vi "MainNR.vi"(10 "JQMHStartup":refnum<class "RQMHStartup.lvclass">, 11 "NewTemplate in":refnum<class "Testing.lvclass">) -> ()   [LabVIEW 2024, in "Testing.lvclass"]
uses:
  Testing.lvclass
  C:/Github/JQMH/JQMHCore/Module/RQMHModule.lvclass
  JQMHCore/JQMHStartup/RQMHStartup.lvclass
  Message Queue_class/RQMHMessageQueue.lvclass/RQMHMessageQueue.ctl
  JQMHCore/Module/InitialiseReplyArgs.ctl
  <vilib>/Utility/miscctls.llb/LVPointTypeDef.ctl
  JQMHCore/Module/RQMHModule.lvclass/RQMHModule.ctl
  Do Something ReplyArgs.ctl
  Do Something Args.ctl
  NewRequest ReplyArgs.ctl
  NewRequest Args.ctl
  JQMHCore/Module/Read ModuleName.vi
  JQMHCore/Module/Read External Start.vi
  Message Queue_class/Delacor_lib_QMH_Enqueue Message (Single).vi
  Message Queue_class/RQMHMessageQueue.lvclass
  Testing.lvclass/Testing.ctl
  JQMHCore/Module/RQMHModule.lvclass
  JQMHCore/Shared/JQMHShared.lvlib
panel:
  out "error out":errorcluster
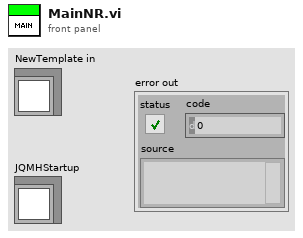
[diagram p1: front panel]
types:
  T1 = typedef "Testing.lvclass/Request Events--cluster.ctl" = cluster{"Do Something":refnum<user-event>, "NewRequest":refnum<user-event>}
  T2 = cluster{"Stop Module":refnum<user-event>, "Requests":T1}
  T3 = typedef "LVPointTypeDef.ctl" = cluster{"Horizontal":i16, "Vertical":i16}
  T4 = enum32{"Invalid", "Standard", "Closed", "Hidden", "Minimized", "Maximized"}
  T5 = typedef "RQMHModule.lvclass/InitialiseReplyArgs.ctl" = cluster{"Did Init?":bool}
  T6 = typedef "Testing.lvclass/Do Something Args.ctl" = cluster{"Msg":string}
  T7 = typedef "Testing.lvclass/Do Something ReplyArgs.ctl" = cluster{"Value":dbl, "Boolean":bool}
  T8 = typedef "Testing.lvclass/NewRequest Args.ctl" = cluster{"String":string}
  T9 = typedef "Testing.lvclass/NewRequest ReplyArgs.ctl" = cluster{"Numeric":dbl}
  T10 = typedef "RQMHModule.lvclass/Reply.ctl" = cluster{"Expects Reply":bool, "Reply":refnum<notifier>}
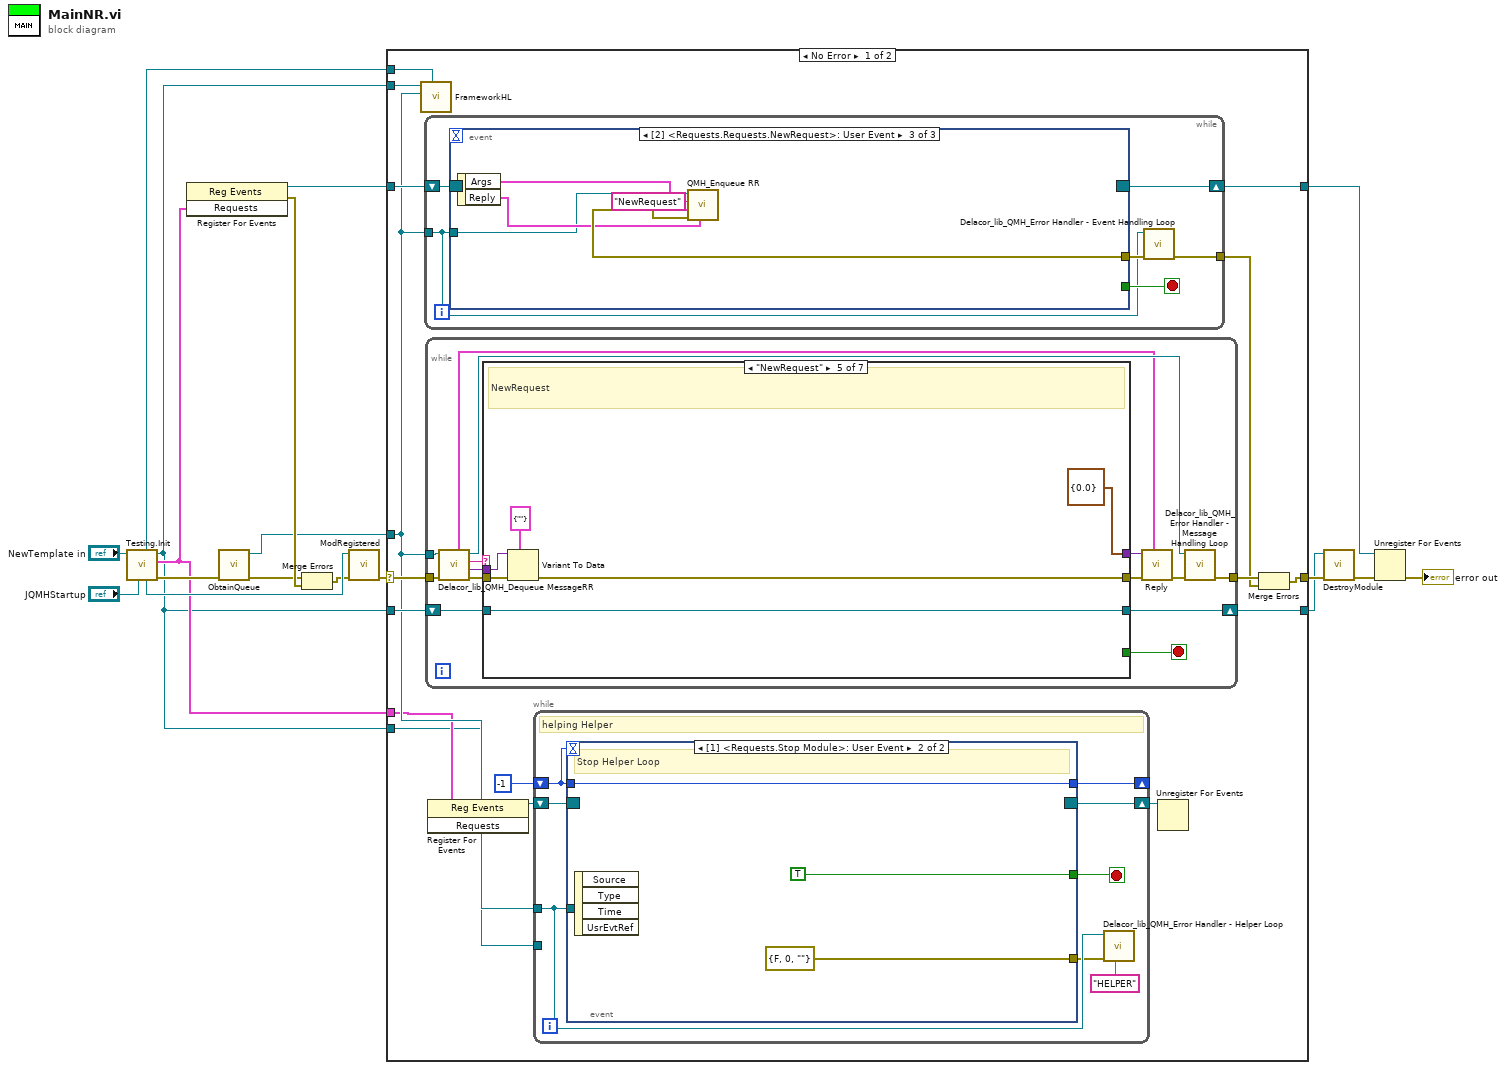
[diagram p0: block diagram]
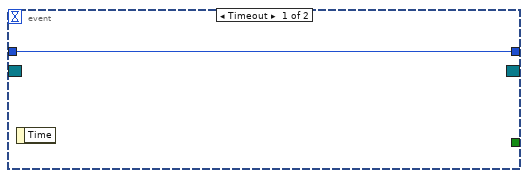
[diagram p2: hidden frame]
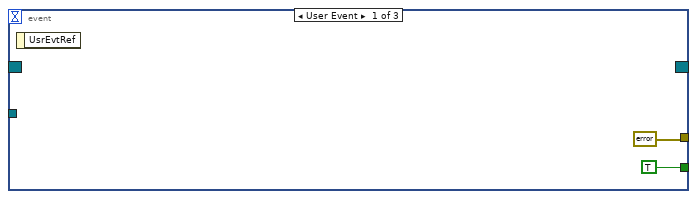
[diagram p3: hidden frame]
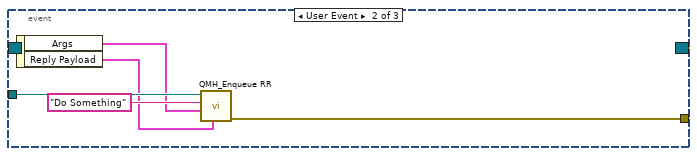
[diagram p4: hidden frame]
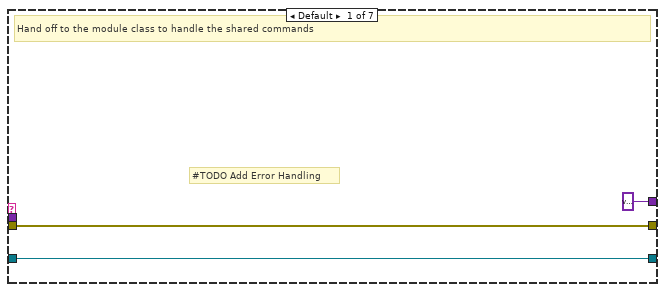
[diagram p5: hidden frame]
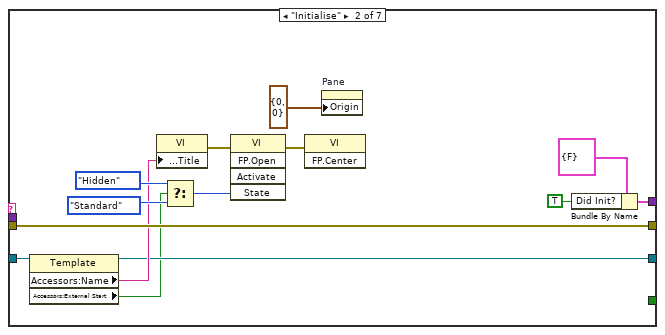
[diagram p6: hidden frame]
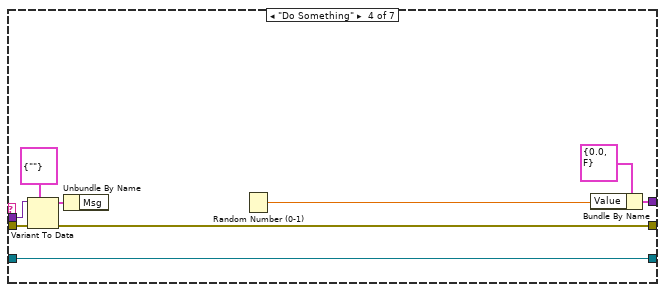
[diagram p8: hidden frame]
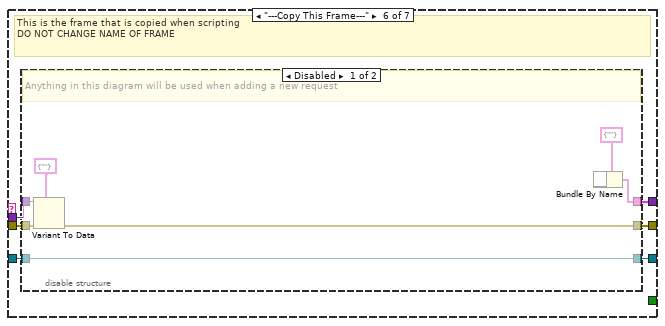
[diagram p9: hidden frame]
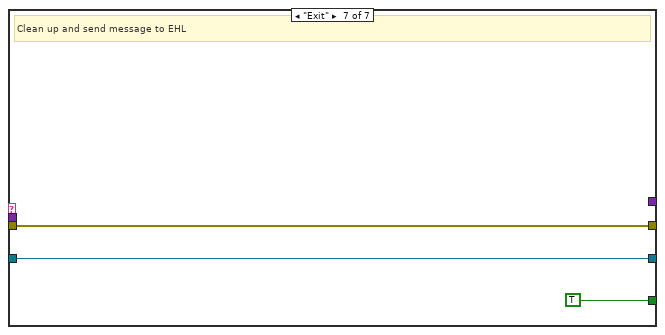
[diagram p11: hidden frame]
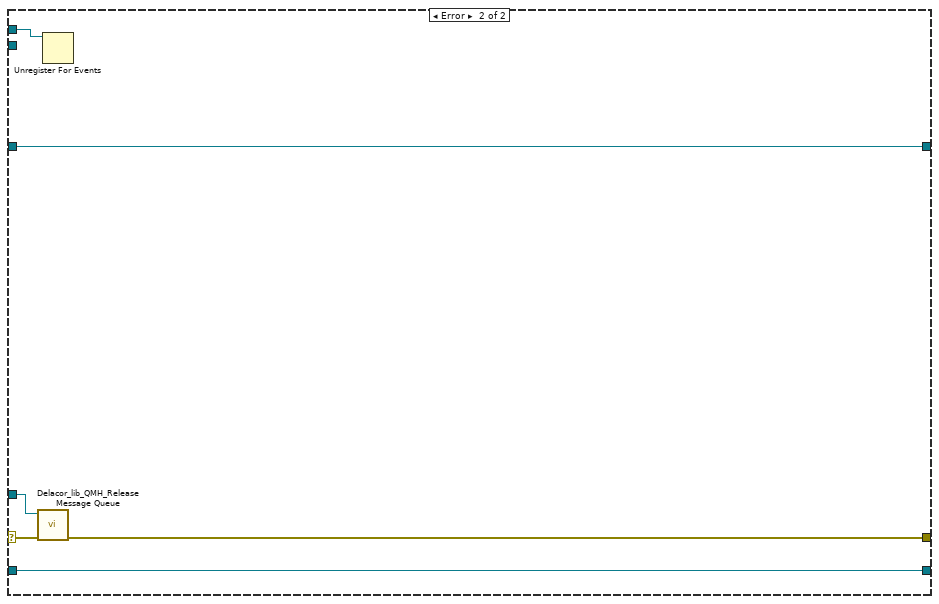
[diagram p12: hidden frame]
diagram:
  n1 = call "Testing.Init.vi"("JQMHStartup in"="JQMHStartup", "NewTemplate in"="NewTemplate in") -> ("error out"=w11:errorcluster, "Requests"=w2:T2, "NewTemplate out"=w1:refnum<class "Testing.lvclass">, "JQMHStartup out"=w9:refnum<class "RQMHStartup.lvclass">, "StandardRequests"=w5:refnum<event-registration>)  [unwired: 4 in, 1 out]
  n2 = register-events(w2) -> (reference out=w4:refnum<event-registration>, error out=w18:errorcluster)  [unwired: 2 in]
  n3 = call "ObtainQueue.vi"("error in"=w11) -> ("error out"=w10:errorcluster, "Message Queue"=w6:refnum<class "RQMHMessageQueue.lvclass">)  [unwired: 9 in]
  n4 = Merge Errors(w10, w18) -> (w7:errorcluster)
  n5 = call "ModRegistered.vi"("error in (no error)"=w7, "JQMHStartup in"=w9) -> ("error out"=w8:errorcluster)  [unwired: 9 in]
  n6 = case "RQMH_MAIN" shown="No Error" w8 {
    selector: w8 -> [w31 w134]
    tunnel: w1 -> [w34 w133]
    tunnel: [w33 w136] -> w17
    tunnel: w4 -> [w32 w136]
    tunnel: w6 -> [w25 w135]
    tunnel: [w30 w133] -> w3
    tunnel: [w27 w132] -> w14
    tunnel: w1 -> [w26 _]
    tunnel: w5 -> [w24 w131]
    tunnel: w2 -> [w23 _]
    tunnel: w1 -> [w22 _]
    frame No Error {
      n7 = call-dynamic "FrameworkHL.vi"("StandardRequests"=w24, "Message Queue"=w25, "JQMHModule in"=w26) -> ()  [unwired: 9 in]
      n8 = while {
        shift-right: [w52] -> w33
        shift-left: w32 -> [w47]
        tunnel: w25 -> [w48]
        tunnel: [w49] -> w28
        stop <- w51 stop-if-true
        n9 = event "RQMH_EVENT_MAIN" shown="[2] <Requests.Requests.NewRequest>: User Event" {
          selector: w47 -> [_ _ _]
          dyn-events: [_ _ _] -> w52
          timeout: _ -> [_ _ _]
          tunnel: [TRUE _ _] -> w51
          tunnel: w48 -> [_ w59 w61]
          tunnel: [errorcluster {"status"=FALSE, "code"=0, "source"=""} ("error out") w56 w64] -> w50
          event User Event {
            n10 = event-data() -> ()  [unwired: 1 in, 1 out]
          }
          event User Event {
            n11 = event-data() -> ("Args"=w57:T6, "Reply Payload"=w55:T10)  [unwired: 1 in]
            n12 = call "QMH_Enqueue RR.vi"("Reply"=w55, "Message Data"=w57, "Message"="Do Something", "Message Queue in"=w59) -> ("error out"=w56:errorcluster)  [unwired: 6 in, 1 out]
          }
          event User Event {
            n13 = event-data() -> ("Args"=w62:T8, "Reply"=w63:T10)  [unwired: 1 in]
            n14 = call "QMH_Enqueue RR.vi"("Reply"=w63, "Message Data"=w62, "Message"="NewRequest", "Message Queue in"=w61) -> ("error out"=w64:errorcluster)  [unwired: 6 in, 1 out]
          }
        }
        n15 = call-dynamic "Delacor_lib_QMH_Error Handler - Event Handling Loop.vi"("error in"=w50, "Message Queue in"=w48) -> ("dup error in"=w49:errorcluster)  [unwired: 8 in, 1 out]
      }
      n16 = while {
        tunnel: w25 -> [w73]
        tunnel: w31 -> [w72]
        shift-right: [w75] -> w30
        shift-left: w34 -> [w76]
        tunnel: [w74] -> w29
        stop <- w78 stop-if-true
        n17 = call-dynamic "Delacor_lib_QMH_Dequeue MessageRR.vi"("error in"=w72, "Message Queue in"=w73) -> ("error out"=w71:errorcluster, "Message Data"=w69:variant, "Message"=w70:string, "Message Queue out"=w77:refnum<class "RQMHMessageQueue.lvclass">, "Reply"=w65:T10)  [unwired: 5 in]
        n18 = case "RQMH_MESSAGE_CASES" shown="\"NewRequest\"" w70 {
          tunnel: [_ _ _ _ _ _ TRUE] -> w78
          tunnel: w76 -> [w80 w83 w96 w106 w110 w116 w129]
          tunnel: w69 -> [_ _ _ w102 w109 w114 _]
          tunnel: w71 -> [w81 w95 w97 w101 w112 w118 w128]
          tunnel: [w81 w95 w97 w100 w111 w117 w128] -> w68
          tunnel: [w80 w84 w96 w106 w110 w115 w129] -> w75
          tunnel: [variant w94 _ w105 T9 {"Numeric"=0.0} ("RQMH_MHL_REPLY_PL") w113 _] -> w66
          frame Default {
            # "#TODO Add Error Handling"
            # "Hand off to the module class to handle the shared commands"
          }
          frame "Initialise" {
            n19 = property class="Template"(reference=w83) -> (reference out=w84:refnum<class "Testing.lvclass">, "Accessors:Name"=w85:string, "Accessors:External Start"=w82:bool)  [unwired: 1 in, 1 out]
            n20 = property on="Property Node" class="VI"("Front Panel.Title"=w85) -> (error out=w92:errorcluster)  [unwired: 2 in, 1 out]
            n21 = Select(t=T4."Hidden" ("State"), s=w82, f=T4."Standard" ("State")) -> (s? t:f=w88:T4)
            n22 = invoke on="Invoke Node" class="VI" method="FP.Open"(error in=w92, "State"=w88) -> (error out=w91:errorcluster)  [unwired: 3 in, 4 out]
            n23 = invoke on="Invoke Node" class="VI" method="FP.Center"(error in=w91) -> ()  [unwired: 2 in, 3 out]
            n24 = property on="Pane" class="Pane"("Origin"=T3 {"Horizontal"=0, "Vertical"=0}) -> ()  [unwired: 2 in, 2 out]
            n25 = Bundle By Name(cluster=T5 {"Did Init?"=FALSE} ("Args"), "Did Init?"=TRUE) -> (w94:T5)
          }
          frame "---Module Specific---" {
          }
          frame "Do Something" {
            n26 = Variant To Data(error in=w101, type=T6 {"Msg"=""} ("Do Something Args"), Variant=w102) -> (data=w98:T6, error out=w100:errorcluster)
            n27 = Unbundle By Name(w98) -> ()  [unwired: 1 out]
            n28 = Random Number (0-1)() -> (number: 0 to 1=w103:dbl)
            n29 = Bundle By Name(cluster=T7 {"Value"=0.0, "Boolean"=FALSE}, "Value"=w103) -> (w105:T7)
          }
          frame "NewRequest" {
            # "NewRequest"
            n30 = Variant To Data(error in=w112, type=T8 {"String"=""} ("RQMH_MHL_MSG_PL"), Variant=w109) -> (error out=w111:errorcluster)  [unwired: 1 out]
          }
          frame "---Copy This Frame---" {
            # "This is the frame that is copied when scripting\nDO NOT CHANGE NAME OF FRAME"
            n31 = disable-structure shown="Disabled" {
              disable-tunnel: w118 -> [w122 w127]
              disable-tunnel: [w123 w127] -> w117
              disable-tunnel: w116 -> [w125 w126]
              disable-tunnel: [w125 w126] -> w115
              disable-tunnel: w114 -> [w124 _]
              disable-tunnel: [w120 _] -> w113
              frame Disabled {
                # "Anything in this diagram will be used when adding a new request"
                n32 = Variant To Data(error in=w122, type=cluster{string} {""} ("RQMH_MHL_MSG_PL"), Variant=w124) -> (error out=w123:errorcluster)  [unwired: 1 out]
                n33 = Bundle By Name(cluster=cluster{string} {""} ("RQMH_MHL_REPLY_PL")) -> (w120:cluster{string})  [unwired: 1 in]
              }
              frame Enabled {
              }
            }
          }
          frame "Exit" {
            # "Clean up and send message to EHL"
          }
        }
        n34 = call "Reply.vi"("Reply"=w65, "error in (no error)"=w68, "ReplyPayload"=w66) -> ("error out"=w67:errorcluster)  [unwired: 8 in]
        n35 = call-dynamic "Delacor_lib_QMH_Error Handler - Message Handling Loop.vi"("error in"=w67, "Message Queue in"=w77) -> ("dup error in"=w74:errorcluster)  [unwired: 8 in, 1 out]
      }
      n36 = register-events ("DQMH_HELPER_REGFOREVENTS")(w23) -> (reference out=w20:refnum<event-registration>)  [unwired: 2 in, 1 out]
      n37 = while "RQMH_HELPER_LOOP" {
        shift-right: [w42] -> _
        shift-left: -1 -> [w41]
        shift-right: [w39] -> w19
        shift-left: w20 -> [w40]
        tunnel: w25 -> [w37]
        tunnel: w22 -> [_]
        stop <- w38 stop-if-true
        # "helping Helper"
        n38 = event "RQMH_HELPER_EVENT_STRUCTURE" shown="[1] <Requests.Stop Module>: User Event" {
          selector: w40 -> [_ _]
          dyn-events: [_ _] -> w39
          timeout: w41 -> [_ _]
          tunnel: w41 -> [w43 w46]
          tunnel: [w43 w46] -> w42
          tunnel: [_ TRUE] -> w38
          tunnel: [_ errorcluster {"status"=FALSE, "code"=0, "source"=""} ("error constant")] -> w35
          tunnel: w37 -> [_ _]
          event Timeout {
            n39 = event-data() -> ()  [unwired: 1 in, 1 out]
          }
          event User Event {
            # "Stop Helper Loop"
            n40 = event-data() -> ()  [unwired: 1 in, 4 out]
          }
        }
        n41 = call-dynamic "Delacor_lib_QMH_Error Handler - Helper Loop.vi"("HelperName"="HELPER" ("RQMH_HELPER_LOOP_NAME"), "error in"=w35, "Message Queue in"=w37) -> ()  [unwired: 7 in, 2 out]
      }
      n42 = Unregister For Events(event registration refnum=w19) -> ()  [unwired: 1 in, 1 out]
      n43 = Merge Errors(w29, w28) -> (w27:errorcluster)
    }
    frame Error {
      n44 = call-dynamic "Delacor_lib_QMH_Release Message Queue.vi"("error in"=w134, "Message Queue"=w135) -> ("error out"=w132:errorcluster)  [unwired: 9 in]
      n45 = Unregister For Events(event registration refnum=w131) -> ()  [unwired: 1 in, 1 out]
    }
  }
  n46 = call "DestroyModule.vi"("error in (no error)"=w14, "JQMHModule in"=w3) -> ("error out"=w16:errorcluster)  [unwired: 9 in]
  n47 = Unregister For Events(event registration refnum=w17, error in=w16) -> (error out=→"error out":errorcluster)
